vi "ELVIS III v1.0 Build MUX Configuration PWM.vi"(11 "Channel":T4) -> (1 "Configuration Bitmask Array":bool[][](array[boolean]), 2 "Configuration BitCode Array":bool[][](array[boolean]), 3 "Channel Reservation List":T1)   [LabVIEW 2021]
uses:
  <vilib>/myRIO/Common/Instrument Driver Framework/myRIO v1.0/PWM/typedefs/PWM Channels Enum.ctl
  <vilib>/myRIO/Common/Instrument Driver Framework/ELVIS III v1.0/Resource Manager/typedefs/ELVIS III v1.0 Channel Reservation List.ctl
  <vilib>/myRIO/Common/Instrument Driver Framework/ELVIS III v1.0/Resource Manager/typedefs/ELVIS III v1.0 Channel Reservation Info.ctl
  <vilib>/myRIO/Common/Instrument Driver Framework/ELVIS III v1.0/Resource Manager/typedefs/ELVIS III v1.0 Connector List.ctl
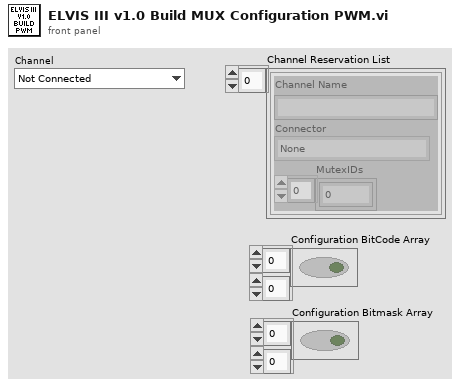
[diagram p1: front panel]
types:
  T1 = typedef "ELVIS III v1.0 Channel Reservation List.ctl" = T2[]
  T2 = typedef "ELVIS III v1.0 Channel Reservation Info.ctl" = cluster{"Channel Name":string, "Connector":T3, "MutexIDs":u32[]}
  T3 = typedef "ELVIS III v1.0 Connector List.ctl" = enum32{"None", "ConnectorA", "ConnectorB"}
  T4 = typedef "PWM Channels Enum.ctl" = enum16{"Not Connected", "C/PWM0", "C/PWM1", "A/PWM0", "A/PWM1", "A/PWM2", "A/PWM3", "A/PWM4", "A/PWM5", "A/PWM6", "A/PWM7", "A/PWM8", "A/PWM9", "A/PWM10", "A/PWM11", "A/PWM12", "A/PWM13", "A/PWM14", "A/PWM15", "A/PWM16", "A/PWM17", "A/PWM18", "A/PWM19", "B/PWM0", "B/PWM1", "B/PWM2", "B/PWM3", "B/PWM4", "B/PWM5", "B/PWM6", "B/PWM7", "B/PWM8", "B/PWM9", "B/PWM10", "B/PWM11", "B/PWM12", "B/PWM13", "B/PWM14", "B/PWM15", "B/PWM16", "B/PWM17", "B/PWM18", "B/PWM19", "PWM/PWM0", "PWM/PWM1", "PWM/PWM2", "PWM/PWM3", "PWM/PWM4", "PWM/PWM5", "PWM/PWM6", "PWM/PWM7", "PWM/PWM8", "PWM/PWM9"}
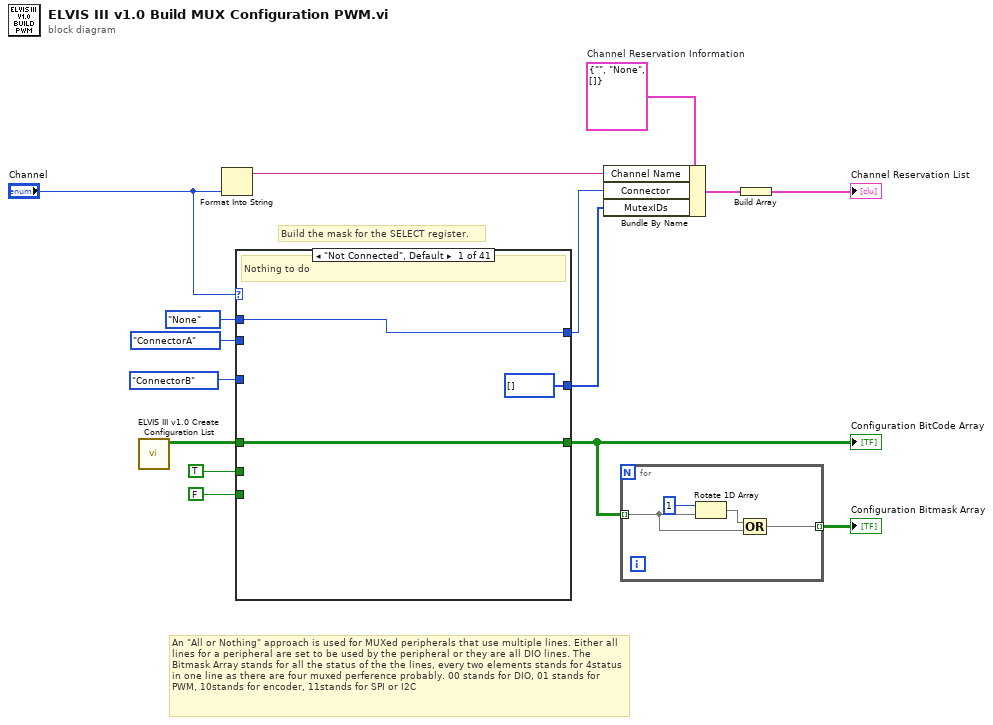
[diagram p0: block diagram]
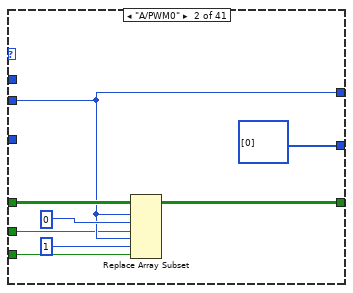
[diagram p2: hidden frame]
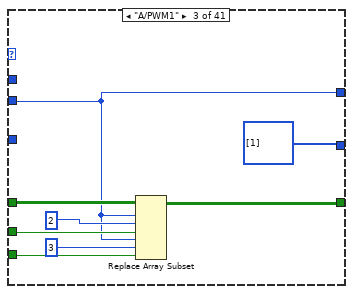
[diagram p3: hidden frame]
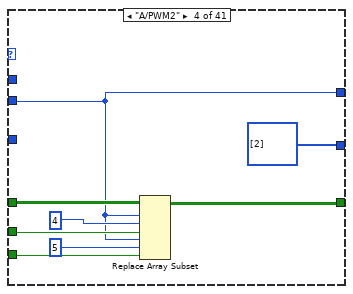
[diagram p4: hidden frame]
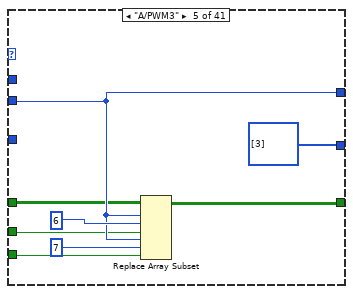
[diagram p5: hidden frame]
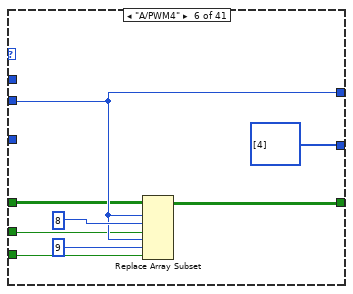
[diagram p6: hidden frame]
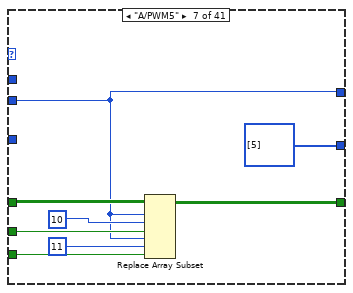
[diagram p7: hidden frame]
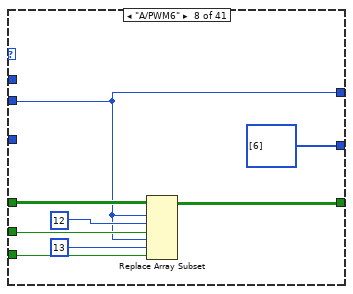
[diagram p8: hidden frame]
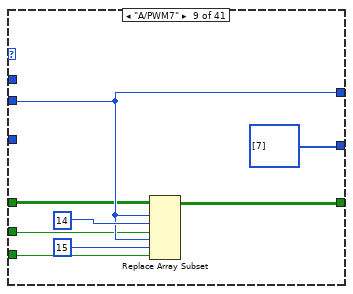
[diagram p9: hidden frame]
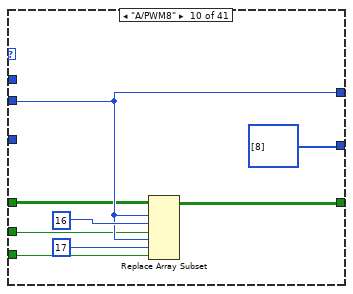
[diagram p10: hidden frame]
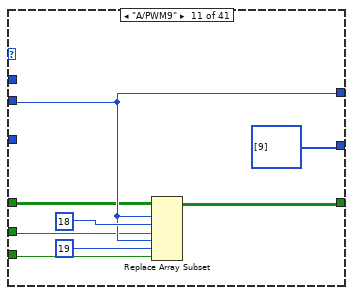
[diagram p11: hidden frame]
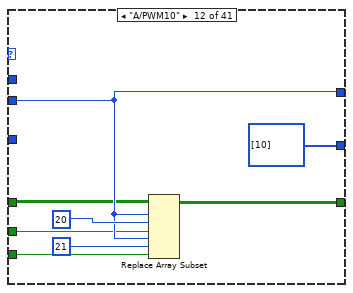
[diagram p12: hidden frame]
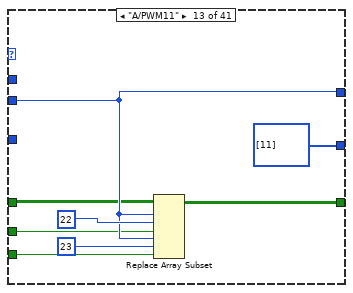
[diagram p13: hidden frame]
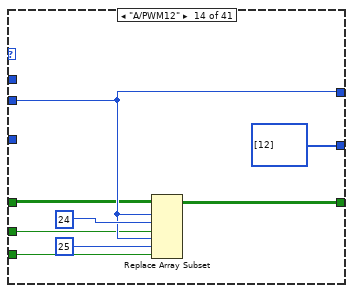
[diagram p14: hidden frame]
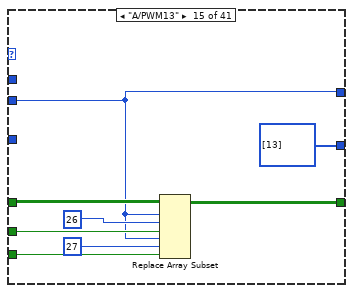
[diagram p15: hidden frame]
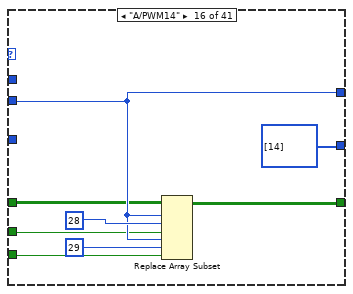
[diagram p16: hidden frame]
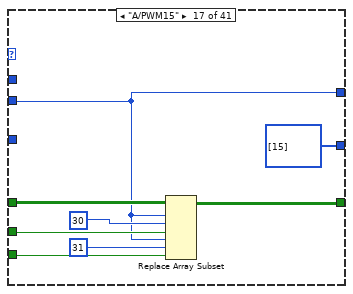
[diagram p17: hidden frame]
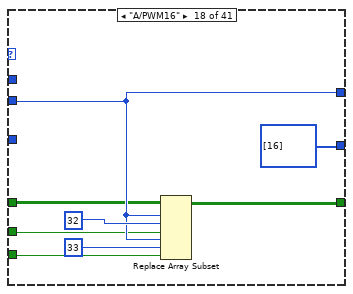
[diagram p18: hidden frame]
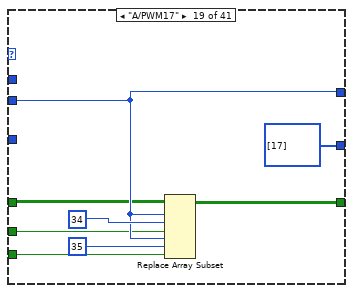
[diagram p19: hidden frame]
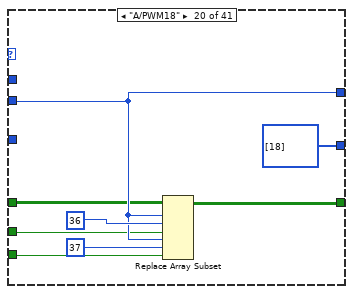
[diagram p20: hidden frame]
diagram:
  w7 = T2 {"Channel Name"="", "Connector"=enum."None", "MutexIDs"=[]}  # Channel Reservation Information
  # "An \"All or Nothing\" approach is used for MUXed peripherals that use multiple lines. Either all lines for a peripheral are set to be used by the peripheral or they are all DIO lines. The Bitmask Array stands for all the status of the the lines, every two elements stands for 4status in one line as there are four muxed perference probably. 00 stands for DIO, 01 stands for PWM, 10stands for encoder, 11stands for SPI or I2C"
  # "Build the mask for the SELECT register."
  n1 = call <vilib>:"ELVIS III v1.0 Create Configuration List.vi"() -> ("Bitmask Array"=w8:bool[][])  [unwired: 11 in]
  n2 = Format Into String("Channel") -> (resulting string=w12:string)  [unwired: 3 in, 1 out]
  n3 = case shown="\"Not Connected\", Default" "Channel" {
    tunnel: w8 -> [w18 w26 w32 w40 w45 w54 w62 w72 w78 w86 w93 w102 w110 w119 w128 w135 w144 w151 w159 w165 w173 w181 w190 w195 w208 w216 w223 w232 w240 w248 w256 w261 w269 w279 w285 w294 w304 w308 w320 w328 w333]
    tunnel: [w18 w22 w29 w36 w47 w55 w61 w69 w77 w87 w94 w103 w109 w116 w125 w132 w141 w150 w156 w166 w174 w182 w187 w196 w205 w213 w220 w229 w239 w245 w253 w262 w270 w278 w286 w292 w301 w307 w317 w323 w334] -> w2
    tunnel: ELVIS_III_v1.0_Connector_List."None" ("Connector List") -> [w17 _ _ _ _ _ _ _ _ _ _ _ _ _ _ _ _ _ _ _ _ _ _ _ _ _ _ _ _ _ _ _ _ _ _ _ _ _ _ _ _]
    tunnel: ELVIS_III_v1.0_Connector_List."ConnectorA" ("Connector List") -> [_ w23 w27 w37 w48 w56 w60 w67 w79 w88 w96 w104 w111 w120 w123 w136 w140 w152 w160 w168 w176 _ _ _ _ _ _ _ _ _ _ _ _ _ _ _ _ _ _ _ _]
    tunnel: TRUE ("new element/subarray") -> [_ w21 w31 w39 w44 w53 w63 w71 w76 w85 w92 w101 w108 w118 w127 w134 w143 w148 w158 w164 w172 w180 w189 w198 w207 w215 w222 w231 w236 w247 w255 w260 w268 w277 w284 w293 w303 w310 w319 w327 w332]
    tunnel: [w17 w23 w27 w37 w48 w56 w60 w67 w79 w88 w96 w104 w111 w120 w123 w136 w140 w152 w160 w168 w176 w184 w191 w200 w203 w212 w224 w227 w237 w244 w251 w264 w272 w280 w288 w295 w300 w312 w315 w325 w336] -> w9
    tunnel: ELVIS_III_v1.0_Connector_List."ConnectorB" ("Connector List") -> [_ _ _ _ _ _ _ _ _ _ _ _ _ _ _ _ _ _ _ _ _ w184 w191 w200 w203 w212 w224 w227 w237 w244 w251 w264 w272 w280 w288 w295 w300 w312 w315 w325 w336]
    tunnel: [u32[] [] u32[] [0] u32[] [1] u32[] [2] u32[] [3] u32[] [4] u32[] [5] u32[] [6] u32[] [7] u32[] [8] u32[] [9] u32[] [10] u32[] [11] u32[] [12] u32[] [13] u32[] [14] u32[] [15] u32[] [16] u32[] [17] u32[] [18] u32[] [19] u32[] [0] u32[] [1] u32[] [2] u32[] [3] u32[] [4] u32[] [5] u32[] [6] u32[] [7] u32[] [8] u32[] [9] u32[] [10] u32[] [11] u32[] [12] u32[] [13] u32[] [14] u32[] [15] u32[] [16] u32[] [17] u32[] [18] u32[] [19]] -> w4
    tunnel: FALSE ("new element/subarray") -> [_ w19 w30 w38 w43 w52 w64 w70 w75 w84 w91 w100 w107 w117 w126 w133 w142 w147 w157 w163 w171 w179 w188 w197 w206 w214 w221 w230 w235 w246 w254 w259 w267 w276 w283 w291 w302 w309 w318 w326 w331]
    frame "Not Connected", Default {
      # "Nothing to do"
    }
    frame "A/PWM0" {
      n4 = Replace Array Subset(array=w26, new element #1=w21, index (row) #1=w23, index (col) #1=0 ("disabled index (col)"), new element #2=w19, index (row) #2=w23, index (col) #2=1 ("disabled index (col)")) -> (w22:bool[][])
    }
    frame "A/PWM1" {
      n5 = Replace Array Subset(array=w32, new element #1=w31, index (row) #1=w27, index (col) #1=2 ("disabled index (col)"), new element #2=w30, index (row) #2=w27, index (col) #2=3 ("disabled index (col)")) -> (w29:bool[][])
    }
    frame "A/PWM2" {
      n6 = Replace Array Subset(array=w40, new element #1=w39, index (row) #1=w37, index (col) #1=4 ("disabled index (col)"), new element #2=w38, index (row) #2=w37, index (col) #2=5 ("disabled index (col)")) -> (w36:bool[][])
    }
    frame "A/PWM3" {
      n7 = Replace Array Subset(array=w45, new element #1=w44, index (row) #1=w48, index (col) #1=6 ("disabled index (col)"), new element #2=w43, index (row) #2=w48, index (col) #2=7 ("disabled index (col)")) -> (w47:bool[][])
    }
    frame "A/PWM4" {
      n8 = Replace Array Subset(array=w54, new element #1=w53, index (row) #1=w56, index (col) #1=8 ("disabled index (col)"), new element #2=w52, index (row) #2=w56, index (col) #2=9 ("disabled index (col)")) -> (w55:bool[][])
    }
    frame "A/PWM5" {
      n9 = Replace Array Subset(array=w62, new element #1=w63, index (row) #1=w60, index (col) #1=10 ("disabled index (col)"), new element #2=w64, index (row) #2=w60, index (col) #2=11 ("disabled index (col)")) -> (w61:bool[][])
    }
    frame "A/PWM6" {
      n10 = Replace Array Subset(array=w72, new element #1=w71, index (row) #1=w67, index (col) #1=12 ("disabled index (col)"), new element #2=w70, index (row) #2=w67, index (col) #2=13 ("disabled index (col)")) -> (w69:bool[][])
    }
    frame "A/PWM7" {
      n11 = Replace Array Subset(array=w78, new element #1=w76, index (row) #1=w79, index (col) #1=14 ("disabled index (col)"), new element #2=w75, index (row) #2=w79, index (col) #2=15 ("disabled index (col)")) -> (w77:bool[][])
    }
    frame "A/PWM8" {
      n12 = Replace Array Subset(array=w86, new element #1=w85, index (row) #1=w88, index (col) #1=16 ("disabled index (col)"), new element #2=w84, index (row) #2=w88, index (col) #2=17 ("disabled index (col)")) -> (w87:bool[][])
    }
    frame "A/PWM9" {
      n13 = Replace Array Subset(array=w93, new element #1=w92, index (row) #1=w96, index (col) #1=18 ("disabled index (col)"), new element #2=w91, index (row) #2=w96, index (col) #2=19 ("disabled index (col)")) -> (w94:bool[][])
    }
    frame "A/PWM10" {
      n14 = Replace Array Subset(array=w102, new element #1=w101, index (row) #1=w104, index (col) #1=20 ("disabled index (col)"), new element #2=w100, index (row) #2=w104, index (col) #2=21 ("disabled index (col)")) -> (w103:bool[][])
    }
    frame "A/PWM11" {
      n15 = Replace Array Subset(array=w110, new element #1=w108, index (row) #1=w111, index (col) #1=22 ("disabled index (col)"), new element #2=w107, index (row) #2=w111, index (col) #2=23 ("disabled index (col)")) -> (w109:bool[][])
    }
    frame "A/PWM12" {
      n16 = Replace Array Subset(array=w119, new element #1=w118, index (row) #1=w120, index (col) #1=24 ("disabled index (col)"), new element #2=w117, index (row) #2=w120, index (col) #2=25 ("disabled index (col)")) -> (w116:bool[][])
    }
    frame "A/PWM13" {
      n17 = Replace Array Subset(array=w128, new element #1=w127, index (row) #1=w123, index (col) #1=26 ("disabled index (col)"), new element #2=w126, index (row) #2=w123, index (col) #2=27 ("disabled index (col)")) -> (w125:bool[][])
    }
    frame "A/PWM14" {
      n18 = Replace Array Subset(array=w135, new element #1=w134, index (row) #1=w136, index (col) #1=28 ("disabled index (col)"), new element #2=w133, index (row) #2=w136, index (col) #2=29 ("disabled index (col)")) -> (w132:bool[][])
    }
    frame "A/PWM15" {
      n19 = Replace Array Subset(array=w144, new element #1=w143, index (row) #1=w140, index (col) #1=30 ("disabled index (col)"), new element #2=w142, index (row) #2=w140, index (col) #2=31 ("disabled index (col)")) -> (w141:bool[][])
    }
    frame "A/PWM16" {
      n20 = Replace Array Subset(array=w151, new element #1=w148, index (row) #1=w152, index (col) #1=32 ("disabled index (col)"), new element #2=w147, index (row) #2=w152, index (col) #2=33 ("disabled index (col)")) -> (w150:bool[][])
    }
    frame "A/PWM17" {
      n21 = Replace Array Subset(array=w159, new element #1=w158, index (row) #1=w160, index (col) #1=34 ("disabled index (col)"), new element #2=w157, index (row) #2=w160, index (col) #2=35 ("disabled index (col)")) -> (w156:bool[][])
    }
    frame "A/PWM18" {
      n22 = Replace Array Subset(array=w165, new element #1=w164, index (row) #1=w168, index (col) #1=36 ("disabled index (col)"), new element #2=w163, index (row) #2=w168, index (col) #2=37 ("disabled index (col)")) -> (w166:bool[][])
    }
    frame "A/PWM19" {
      n23 = Replace Array Subset(array=w173, new element #1=w172, index (row) #1=w176, index (col) #1=38 ("disabled index (col)"), new element #2=w171, index (row) #2=w176, index (col) #2=39 ("disabled index (col)")) -> (w174:bool[][])
    }
    frame "B/PWM0" {
      n24 = Replace Array Subset(array=w181, new element #1=w180, index (row) #1=w184, index (col) #1=0 ("disabled index (col)"), new element #2=w179, index (row) #2=w184, index (col) #2=1 ("disabled index (col)")) -> (w182:bool[][])
    }
    frame "B/PWM1" {
      n25 = Replace Array Subset(array=w190, new element #1=w189, index (row) #1=w191, index (col) #1=2 ("disabled index (col)"), new element #2=w188, index (row) #2=w191, index (col) #2=3 ("disabled index (col)")) -> (w187:bool[][])
    }
    frame "B/PWM2" {
      n26 = Replace Array Subset(array=w195, new element #1=w198, index (row) #1=w200, index (col) #1=4 ("disabled index (col)"), new element #2=w197, index (row) #2=w200, index (col) #2=5 ("disabled index (col)")) -> (w196:bool[][])
    }
    frame "B/PWM3" {
      n27 = Replace Array Subset(array=w208, new element #1=w207, index (row) #1=w203, index (col) #1=6 ("disabled index (col)"), new element #2=w206, index (row) #2=w203, index (col) #2=7 ("disabled index (col)")) -> (w205:bool[][])
    }
    frame "B/PWM4" {
      n28 = Replace Array Subset(array=w216, new element #1=w215, index (row) #1=w212, index (col) #1=8 ("disabled index (col)"), new element #2=w214, index (row) #2=w212, index (col) #2=9 ("disabled index (col)")) -> (w213:bool[][])
    }
    frame "B/PWM5" {
      n29 = Replace Array Subset(array=w223, new element #1=w222, index (row) #1=w224, index (col) #1=10 ("disabled index (col)"), new element #2=w221, index (row) #2=w224, index (col) #2=11 ("disabled index (col)")) -> (w220:bool[][])
    }
    frame "B/PWM6" {
      n30 = Replace Array Subset(array=w232, new element #1=w231, index (row) #1=w227, index (col) #1=12 ("disabled index (col)"), new element #2=w230, index (row) #2=w227, index (col) #2=13 ("disabled index (col)")) -> (w229:bool[][])
    }
    frame "B/PWM7" {
      n31 = Replace Array Subset(array=w240, new element #1=w236, index (row) #1=w237, index (col) #1=14 ("disabled index (col)"), new element #2=w235, index (row) #2=w237, index (col) #2=15 ("disabled index (col)")) -> (w239:bool[][])
    }
    frame "B/PWM8" {
      n32 = Replace Array Subset(array=w248, new element #1=w247, index (row) #1=w244, index (col) #1=16 ("disabled index (col)"), new element #2=w246, index (row) #2=w244, index (col) #2=17 ("disabled index (col)")) -> (w245:bool[][])
    }
    frame "B/PWM9" {
      n33 = Replace Array Subset(array=w256, new element #1=w255, index (row) #1=w251, index (col) #1=18 ("disabled index (col)"), new element #2=w254, index (row) #2=w251, index (col) #2=19 ("disabled index (col)")) -> (w253:bool[][])
    }
    frame "B/PWM10" {
      n34 = Replace Array Subset(array=w261, new element #1=w260, index (row) #1=w264, index (col) #1=20 ("disabled index (col)"), new element #2=w259, index (row) #2=w264, index (col) #2=21 ("disabled index (col)")) -> (w262:bool[][])
    }
    frame "B/PWM11" {
      n35 = Replace Array Subset(array=w269, new element #1=w268, index (row) #1=w272, index (col) #1=22 ("disabled index (col)"), new element #2=w267, index (row) #2=w272, index (col) #2=23 ("disabled index (col)")) -> (w270:bool[][])
    }
    frame "B/PWM12" {
      n36 = Replace Array Subset(array=w279, new element #1=w277, index (row) #1=w280, index (col) #1=24 ("disabled index (col)"), new element #2=w276, index (row) #2=w280, index (col) #2=25 ("disabled index (col)")) -> (w278:bool[][])
    }
    frame "B/PWM13" {
      n37 = Replace Array Subset(array=w285, new element #1=w284, index (row) #1=w288, index (col) #1=26 ("disabled index (col)"), new element #2=w283, index (row) #2=w288, index (col) #2=27 ("disabled index (col)")) -> (w286:bool[][])
    }
    frame "B/PWM14" {
      n38 = Replace Array Subset(array=w294, new element #1=w293, index (row) #1=w295, index (col) #1=28 ("disabled index (col)"), new element #2=w291, index (row) #2=w295, index (col) #2=29 ("disabled index (col)")) -> (w292:bool[][])
    }
    frame "B/PWM15" {
      n39 = Replace Array Subset(array=w304, new element #1=w303, index (row) #1=w300, index (col) #1=30 ("disabled index (col)"), new element #2=w302, index (row) #2=w300, index (col) #2=31 ("disabled index (col)")) -> (w301:bool[][])
    }
    frame "B/PWM16" {
      n40 = Replace Array Subset(array=w308, new element #1=w310, index (row) #1=w312, index (col) #1=32 ("disabled index (col)"), new element #2=w309, index (row) #2=w312, index (col) #2=33 ("disabled index (col)")) -> (w307:bool[][])
    }
    frame "B/PWM17" {
      n41 = Replace Array Subset(array=w320, new element #1=w319, index (row) #1=w315, index (col) #1=34 ("disabled index (col)"), new element #2=w318, index (row) #2=w315, index (col) #2=35 ("disabled index (col)")) -> (w317:bool[][])
    }
    frame "B/PWM18" {
      n42 = Replace Array Subset(array=w328, new element #1=w327, index (row) #1=w325, index (col) #1=36 ("disabled index (col)"), new element #2=w326, index (row) #2=w325, index (col) #2=37 ("disabled index (col)")) -> (w323:bool[][])
    }
    frame "B/PWM19" {
      n43 = Replace Array Subset(array=w333, new element #1=w332, index (row) #1=w336, index (col) #1=38 ("disabled index (col)"), new element #2=w331, index (row) #2=w336, index (col) #2=39 ("disabled index (col)")) -> (w334:bool[][])
    }
  }
  "Configuration BitCode Array" <- w2
  n44 = Bundle By Name(cluster=w7, "Channel Name"=w12, "Connector"=w9, "MutexIDs"=w4) -> (w11:T2)
  n45 = for {
    tunnel: w2 -> [w340] mode=indexing
    tunnel: [w339] -> w1 mode=indexing
    n46 = Rotate 1D Array(1:w340, 2:1 ("n")) -> (0:w341:bool[])
    n47 = Compound Arithmetic op=OR(w341, w340) -> (w339:bool[])
  }
  "Configuration Bitmask Array" <- w1
  n48 = Build Array(w11) -> (→"Channel Reservation List":T2[])
